vi "User Dialog.vi"(8 "error in (no error)":errorcluster, 9 "Timeout (seconds)":dbl=1000.0, 10 "Message":string, 11 "Title":string) -> (0 "error out":errorcluster)   [LabVIEW 2020]
panel:
  in  "Continue":bool
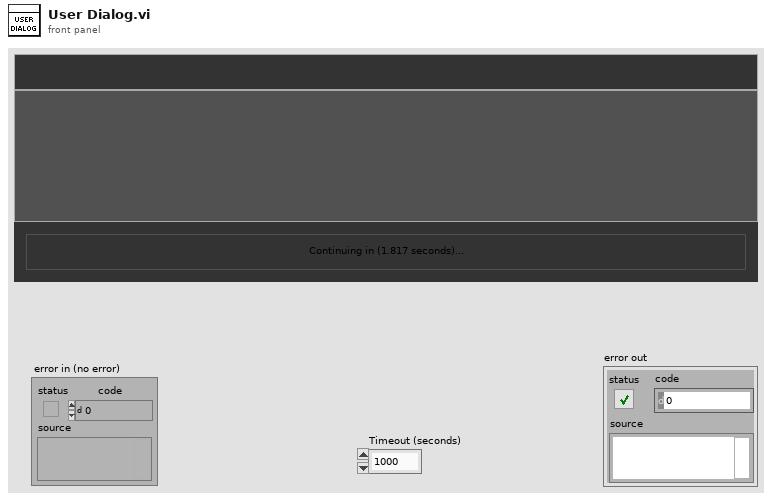
[diagram p1: front panel]
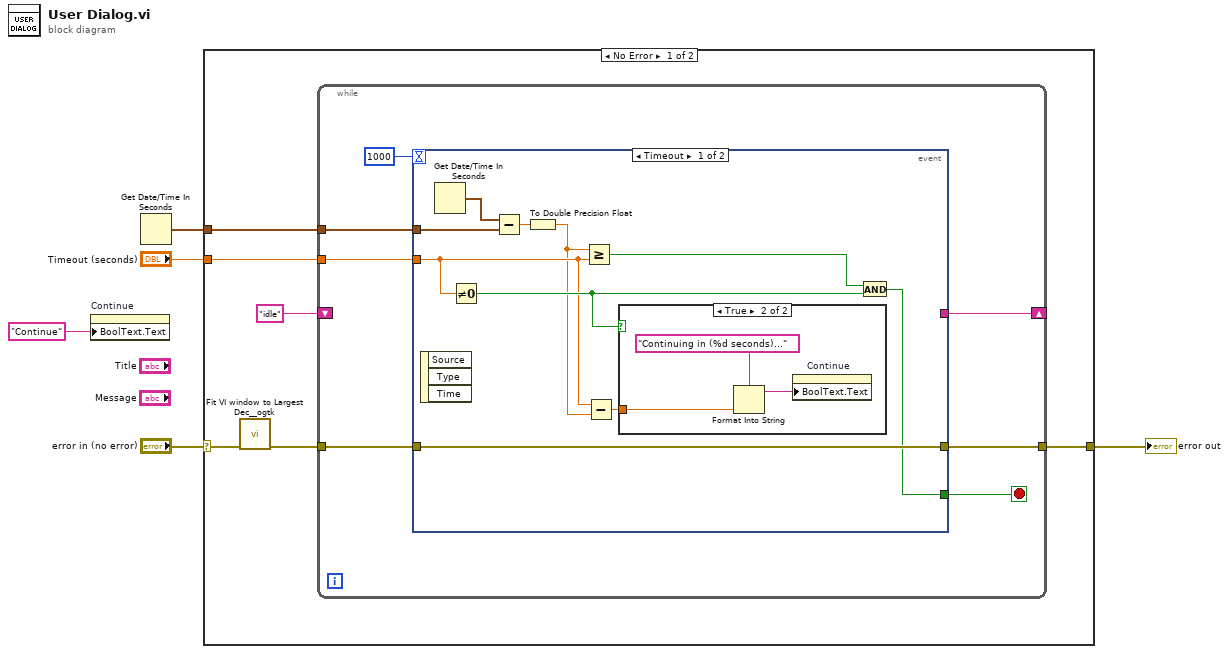
[diagram p0: block diagram]
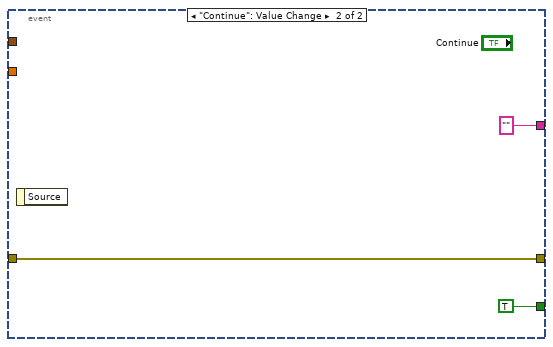
[diagram p3: hidden frame]
diagram:
  n1 = property on="Continue" class="Bool"("BoolText.Text"="Continue" ("Boolean Text.Text")) -> ()  [unwired: 2 in, 2 out]
  n2 = Get Date/Time In Seconds() -> (seconds since 1Jan1904=w3:timestamp)
  n3 = case shown="No Error" "error in (no error)" {
    selector: "error in (no error)" -> [w8 w35]
    tunnel: [w9 w35] -> w5
    tunnel: w3 -> [w7 _]
    tunnel: "Timeout (seconds)" -> [w6 _]
    frame No Error {
      n4 = call <userlib>:"Fit VI window to Largest Dec__ogtk.vi"("error in (no error)"=w8) -> ("error out"=w11:errorcluster)  [unwired: 5 in, 1 out]
      n5 = while {
        tunnel: w11 -> [w18]
        shift-right: [w15] -> _
        shift-left: "idle" -> [_]
        tunnel: [w17] -> w9
        tunnel: w7 -> [w14]
        tunnel: w6 -> [w13]
        stop <- w16 stop-if-true
        n6 = event shown="[0] Timeout" {
          selector: _ -> [_ _]
          dyn-events: _ -> [_ _]
          timeout: 1000 -> [_ _]
          tunnel: w18 -> [w25 w34]
          tunnel: [w25 w34] -> w17
          tunnel: [w23 TRUE] -> w16
          tunnel: [_ ""] -> w15
          tunnel: w14 -> [w27 _]
          tunnel: w13 -> [w20 _]
          event Timeout {
            n7 = event-data() -> ()  [unwired: 1 in, 3 out]
            n8 = Get Date/Time In Seconds() -> (seconds since 1Jan1904=w28:timestamp)
            n9 = Not Equal To 0?(x=w20) -> (x != 0?=w22:bool)
            n10 = Subtract(x=w28, y=w27) -> (x-y=w26:dbl)
            n11 = To Double Precision Float(number=w26) -> (double precision float=w19:dbl)
            n12 = Greater Or Equal?(x=w19, y=w20) -> (x >= y?=w24:bool)
            n13 = Subtract(x=w20, y=w19) -> (x-y=w21:dbl)
            n14 = case shown="True" w22 {
              tunnel: w21 -> [_ w29]
              frame False {
              }
              frame True {
                n15 = Format Into String(format string="Continuing in (%d seconds)...", w29) -> (resulting string=w30:string)  [unwired: 2 in, 1 out]
                n16 = property on="Continue" class="Bool"("BoolText.Text"=w30) -> ()  [unwired: 2 in, 2 out]
              }
            }
            n17 = And(x=w24, y=w22) -> (x .and. y?=w23:bool)
          }
          event "Continue": Value Change {
            n18 = event-data() -> ()  [unwired: 1 in, 1 out]
          }
        }
      }
    }
    frame Error {
    }
  }
  "error out" <- w5
